vi "Config-Chan-SMU-Sampling.vi"(0 "VISA resource name in":refnum<visa-resource-name>, 1 "function":bool, 2 "series resistance *":i32(slide) max=3 scale=0.0..3.0, 5 "unit to configure":i32(slide) max=5 scale=0.0..5.0, 7 "V name (max 6 chars)":string, 9 "standby":bool, 11 "error in (no error)":errorcluster, 12 "mode":i32(slide) max=2 scale=0.0..2.0, 13 "I name (max 6 chars)":string) -> (4 "VISA resource name out":refnum<visa-resource-name>, 15 "error out":errorcluster)   [LabVIEW 2016, in "Agilent 415X Series.lvlib"]
doc: "This VI configures an SMU for SAMPLING mode measurement. \n\nThis VI corresponds to the Channel Definition Page of the instrument (when Measurement Mode is SAMPLING). In general, it allows every setting change that can be made via the instrument's front panel although the change may cause a setting conflict when a measurement is initialied. This VI doesnot allow (by reporting an error) setting changes that can not be made via the instrument's front panel. For example, you may not set Series Resistance for units other than SMU1, SMU2/5.\n\n** The instrument used in the development of this instrument driver does not have an Expander Unit installed. Therefore commands related to SMU5/6 have not been verified."
uses:
  Agilent 415X Series.lvlib
panel:
  # "*    The Series Resistance control is active only for SMU1/2/5(see description)\n**  This VI does NOT report all setting errors.  \n*** Error checking must be done when a measurement is initialized."
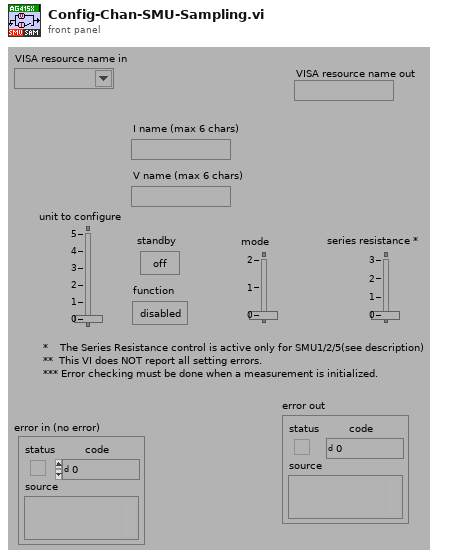
[diagram p1: front panel]
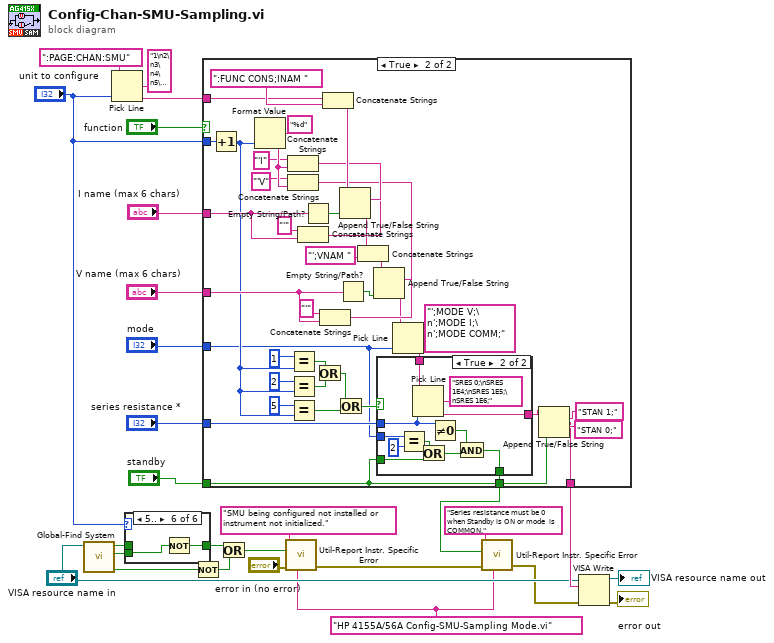
[diagram p0: block diagram]
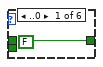
[diagram p2: hidden frame]
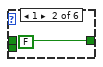
[diagram p3: hidden frame]
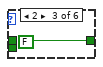
[diagram p4: hidden frame]
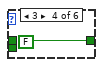
[diagram p5: hidden frame]
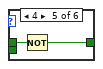
[diagram p6: hidden frame]
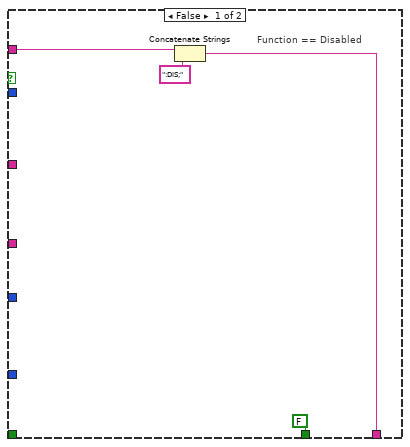
[diagram p7: hidden frame]
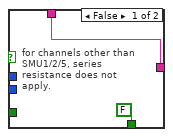
[diagram p8: hidden frame]
diagram:
  w12 = "HP 4155A/56A Config-SMU-Sampling Mode.vi"
  n1 = call "Global-Find System.vi"("VISA session"="VISA resource name in") -> ("found"=w3:bool, "SMU6 present"=w18:bool, "SMU5 present"=w14:bool)  [unwired: 3 in, 5 out]
  n2 = Pick Line(string ("")=":PAGE:CHAN:SMU", multi-line string="1\n2\n3\n4\n5\n6", line index="unit to configure") -> (output string=w25:string)
  n3 = case shown="5.." "unit to configure" {
    tunnel: [FALSE FALSE FALSE FALSE w33 w35] -> w5
    tunnel: w18 -> [_ _ _ _ _ w34]
    tunnel: w14 -> [_ _ _ _ w32 _]
    frame ..0 {
    }
    frame 1 {
    }
    frame 2 {
    }
    frame 3 {
    }
    frame 4 {
      n4 = Not(x=w32) -> (.not. x?=w33:bool)
    }
    frame 5.. {
      n5 = Not(x=w34) -> (.not. x?=w35:bool)
    }
  }
  n6 = Not(x=w3) -> (.not. x?=w2:bool)
  n7 = case shown="True" "function" {
    tunnel: w25 -> [w39 w40]
    tunnel: "unit to configure" -> [_ w48]
    tunnel: "I name (max 6 chars)" -> [_ w73]
    tunnel: "V name (max 6 chars)" -> [_ w64]
    tunnel: "mode" -> [_ w43]
    tunnel: "series resistance *" -> [_ w57]
    tunnel: "standby" -> [_ w44]
    tunnel: [w37 w45] -> w21
    tunnel: [FALSE w42] -> w10
    frame False {
      # "Function == Disabled"
      n8 = Concatenate Strings(w39, ":DIS;") -> (w37:string)
    }
    frame True {
      n9 = Increment(x=w48) -> (x+1=w46:i32)
      n10 = Format Value(format string="%d", value (0)=w46) -> (output string=w77:string)  [unwired: 1 in]
      n11 = Concatenate Strings("'I", w77) -> (w74:string)
      n12 = Concatenate Strings("'V", w77) -> (w67:string)
      n13 = Equal?(x=1, y=w46) -> (x = y?=w53:bool)
      n14 = Equal?(x=2, y=w46) -> (x = y?=w52:bool)
      n15 = Equal?(x=5, y=w46) -> (x = y?=w51:bool)
      n16 = Concatenate Strings("'", w73) -> (w71:string)
      n17 = Empty String/Path?(string/path=w73) -> (empty?=w79:bool)
      n18 = Or(x=w53, y=w52) -> (x .or. y?=w50:bool)
      n19 = Concatenate Strings("'", w64) -> (w63:string)
      n20 = Concatenate Strings(w40, ":FUNC CONS;INAM ") -> (w80:string)
      n21 = Or(x=w50, y=w51) -> (x .or. y?=w49:bool)
      n22 = Empty String/Path?(string/path=w64) -> (empty?=w66:bool)
      n23 = Append True/False String(1:w79, 2:w71, 3:w74, 4:w80) -> (0:w70:string)
      n24 = Concatenate Strings(w70, "';VNAM ") -> (w68:string)
      n25 = Append True/False String(1:w66, 2:w63, 3:w67, 4:w68) -> (0:w61:string)
      n26 = Pick Line(string ("")=w61, multi-line string="';MODE V;\n';MODE I;\n';MODE COMM;", line index=w43) -> (output string=w58:string)
      n27 = case shown="True" w49 {
        tunnel: w58 -> [w82 w92]
        tunnel: w57 -> [_ w85]
        tunnel: [w82 w91] -> w56
        tunnel: w44 -> [_ w88]
        tunnel: w43 -> [_ w90]
        tunnel: [FALSE w83] -> w42
        frame False {
          # "for channels other than\nSMU1/2/5, series \nresistance does not \napply."
        }
        frame True {
          n28 = Equal?(x=w90, y=2) -> (x = y?=w87:bool)
          n29 = Pick Line(string ("")=w92, multi-line string="SRES 0;\nSRES 1E4;\nSRES 1E5;\nSRES 1E6;", line index=w85) -> (output string=w91:string)
          n30 = Or(x=w87, y=w88) -> (x .or. y?=w86:bool)
          n31 = Not Equal To 0?(x=w85) -> (x != 0?=w84:bool)
          n32 = And(x=w84, y=w86) -> (x .and. y?=w83:bool)
        }
      }
      n33 = Append True/False String(1:w44, 2:"STAN 0;", 3:"STAN 1;", 4:w56) -> (0:w45:string)
    }
  }
  n34 = Or(x=w5, y=w2) -> (x .or. y?=w4:bool)
  n35 = call "Util-Report Instr. Specific Error.vi"("source"=w12, "error in (no error)"="error in (no error)", "error message"="SMU being configured not installed or instrument not initialized.", "new error"=w4) -> ("error out"=w8:errorcluster)  [unwired: 6 in, 1 out]
  n36 = call "Util-Report Instr. Specific Error.vi"("source"=w12, "error in (no error)"=w8, "error message"="Series resistance must be 0 when Standby is ON or mode  is COMMON.", "new error"=w10) -> ("error out"=w9:errorcluster)  [unwired: 6 in, 1 out]
  n37 = VISA Write(VISA resource name="VISA resource name in", write buffer=w21, error in (no error)=w9) -> (VISA resource name out=→"VISA resource name out":refnum<visa-resource-name>, error out=→"error out":errorcluster)  [unwired: 1 out]
